vi "DC_Bus_v1.vi"(10 "Control Board VISA":refnum<visa-resource-name>, 11 "HMP4040 VISA":refnum<visa-resource-name>) -> (0 "INV B (10V)":dbl, 1 "INV A (10V)":dbl, 2 "INV B (0V)":dbl, 3 "INV A (0V)":dbl)   [LabVIEW 2019]
uses:
  Ctls/ADC_Select_v1.ctl
  Ctls/Powersupply_Auto_Enum_v1.ctl
panel:
  out "Inv_DC":dbl[](array[numeric])
  out "error out":errorcluster
  in  "error in (no error)":errorcluster
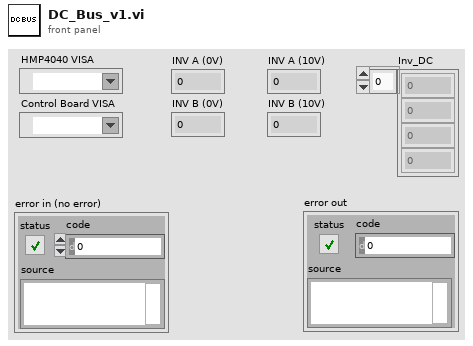
[diagram p1: front panel]
types:
  T1 = typedef "Powersupply_Auto_Enum_v1.ctl" = enum16{"Off", "Control Power", "HMP2020 Control + DC32V", "HMP2020 Control + DC8V", "HMP4040 Control + DC32V", "HMP4040 Control +DC8V"}
  T2 = typedef "ADC_Select_v1.ctl" = enum16{"INVA_ISENSE_U", "INVA_ISENSE_V", "INVA_ISENSE_W", "INVA_UDC", "INVA_TEMP", "HB_TEMP", "AUXB_TEMP", "VLINE_AB", "VLINE_BC", "VLINE_CA", "VSENSE_POS_24V", "VSENSE_POS_5V", "VSENSE_NEG_15V", "INVB_ISENSE_U", "INV_B_ISENSEV", "INVB_ISENSE_W", "INVB_UDC", "INVB_TEMP", "AUXA_TEMP", "AUXC_TEMP", "VOUT_AB", "VOUT_BC", "VOUT_CA", "VSENSE_POS_15V", "VSENSE_POS_3P3V", "TEST_POINT"}
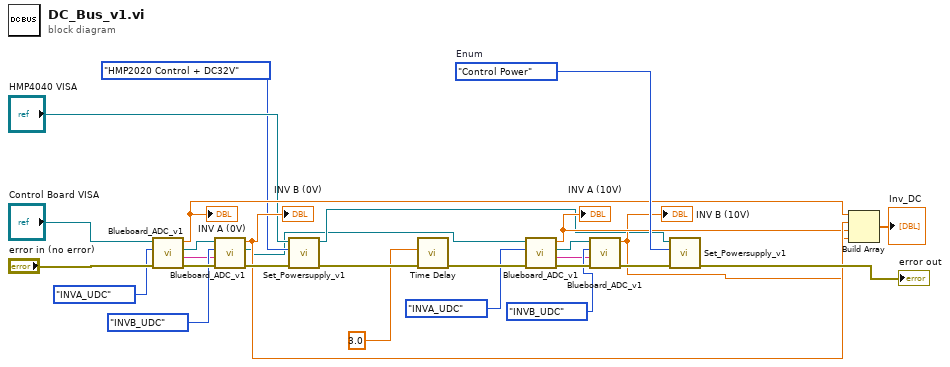
[diagram p0: block diagram]
diagram:
  w18 = Powersupply_Auto_Enum_v1."Control Power"  # Enum
  n1 = call "Blueboard_ADC_v1.vi"("error in (no error)"="error in (no error)", "Blue Board Enum"=ADC_Select_v1."INVA_UDC", "ControlBoard VISA"="Control Board VISA") -> ("error out"=w27:errorcluster, "Message OUT"=w2:string, "VISA Refnum out"=w5:refnum<visa-resource-name>, "Result"=w17:dbl)  [unwired: 5 in]
  "INV A (0V)" <- w17
  n2 = call "Blueboard_ADC_v1.vi"("error in (no error)"=w27, "Message IN"=w2, "Blue Board Enum"=ADC_Select_v1."INVB_UDC", "ControlBoard VISA"=w5) -> ("error out"=w26:errorcluster, "VISA Refnum out"=w4:refnum<visa-resource-name>, "Result"=w16:dbl)  [unwired: 4 in, 1 out]
  "INV B (0V)" <- w16
  n3 = call "Set_Powersupply_v1.vi"("error in (no error)"=w26, "Enum"=Powersupply_Auto_Enum_v1."HMP2020 Control + DC32V", "HMP VISA"="HMP4040 VISA") -> ("error out"=w28:errorcluster, "HMP VISA Out"=w6:refnum<visa-resource-name>)  [unwired: 7 in]
  n4 = call "Time Delay"("error in (no error)"=w28, "Delay Time (s)"=3.0) -> ("error out"=w24:errorcluster)  [unwired: 9 in]
  n5 = call "Blueboard_ADC_v1.vi"("error in (no error)"=w24, "Blue Board Enum"=ADC_Select_v1."INVA_UDC", "ControlBoard VISA"=w4) -> ("error out"=w25:errorcluster, "Message OUT"=w1:string, "VISA Refnum out"=w3:refnum<visa-resource-name>, "Result"=w15:dbl)  [unwired: 5 in]
  "INV A (10V)" <- w15
  n6 = call "Blueboard_ADC_v1.vi"("error in (no error)"=w25, "Message IN"=w1, "Blue Board Enum"=ADC_Select_v1."INVB_UDC", "ControlBoard VISA"=w3) -> ("error out"=w22:errorcluster, "Result"=w14:dbl)  [unwired: 4 in, 2 out]
  "INV B (10V)" <- w14
  n7 = call "Set_Powersupply_v1.vi"("error in (no error)"=w22, "Enum"=w18, "HMP VISA"=w6) -> ("error out"=→"error out":errorcluster)  [unwired: 7 in, 1 out]
  n8 = Build Array(w17, w16, w15, w14) -> (→"Inv_DC":dbl[])
